vi "configure.vi"(8 "error in (no error)":errorcluster, 11 "DL090202ScanHead in":refnum<class "ScanHeadDL090202.lvclass">) -> (0 "error out":errorcluster, 3 "DL090202ScanHead out":refnum<class "ScanHeadDL090202.lvclass">)   [LabVIEW 2010, in "ScanHeadDL090202.lvclass"]
uses:
  ScanHeadDL090202.lvclass
  common/xcontrols/XComponentSpecification/XComponentSpecification/XComponentSpecification.xctl
  common/clusters/plugin_specification.ctl
  SignalWriter/GenericSignalWriter/GenericSignalWriter/GenericSignalWriter.lvclass
  ScanHeadDL090202.lvclass/ScanHeadDL090202.ctl
  Clock/GenericClock/GenericClock/GenericClock.lvclass
  DigitalOut/GenericDigitalOut/GenericDigitalOut/GenericDigitalOut.lvclass
  common/classes/ErrorController/ErrorController/class_data.vi
  common/classes/GenericComponent/GenericComponent/GenericComponent.lvclass
  common/classes/ErrorController/ErrorController/ErrorController.lvclass
panel:
  out "Configuration":string
  in  "cancel":bool
  in  "save":bool
  in  "Tab Control":T1(tab)=enum."shutter digital output"
  in  "x scanner factor":dbl[unit]=1000000.0 caption="translation factor"
  in  "y scanner factor":dbl[unit]=1000000.0 caption="translation factor"
  in  "z scanner factor":dbl[unit]=1000000.0 caption="translation factor"
  in  "xScanner spec":T2(xcontrol)
  in  "yScanner spec":T2(xcontrol)
  in  "zScanner spec":T2(xcontrol)
  in  "modifier factor":dbl=1.0 caption="translation factor"
  in  "intensity modified spec":T2(xcontrol)
  in  "clock spec":T2(xcontrol)
  in  "shutter digitalOut spec":T2(xcontrol)
  in  "offset Z":bool
  in  "offset Y":bool
  in  "offset X":bool
  in  "rotate Z":bool
  in  "zoom":bool
  in  "rotate X":bool
  # "Configure ScanHeadDL090202"
  # "SignalWriter components generate actuator values send to the scanners, each scanner has its own signal writer component.\n\nTranslation factors specify how the trajectory coordinates, which are defined in um space, are translated into the voltage values that are provided to the signalWriter component for each scanner."
  # "x scanner"
  # "y scanner"
  # "z scanner"
  # "Each pixel of the trajectory has a corresponding intensity value. Like the scanner values, the intensity control signal is generated by a SignalWriter component.\n\nThe translation factor specifies how an intensity value is translated into a voltage that is provided to the intensity modifier (such as a pockels cell).\nExample: 100% should correspond to 1.00V provided to a Pockels cell modulator; this would require the translation factor to be 0.01."
  # "The pixel clock is a Clock component that generates the TTL signal that is timingthe SignalWriter components generating the scanner and intensity modulator control signal."
  # "Here you can specify a software-controlled laser shutter. In case you are using an FPGA integrator, we recommend to use the shutter output of the Hifo ADC, because it is faster and more reliable. Leave empty in that case."
  # "Which user interface controls shall be visible?"
  # "For some sophisticated line-scan imagingModes, zooming and rotating etc. doesn't make sense, so the corresponding GUI controls should not be visible."
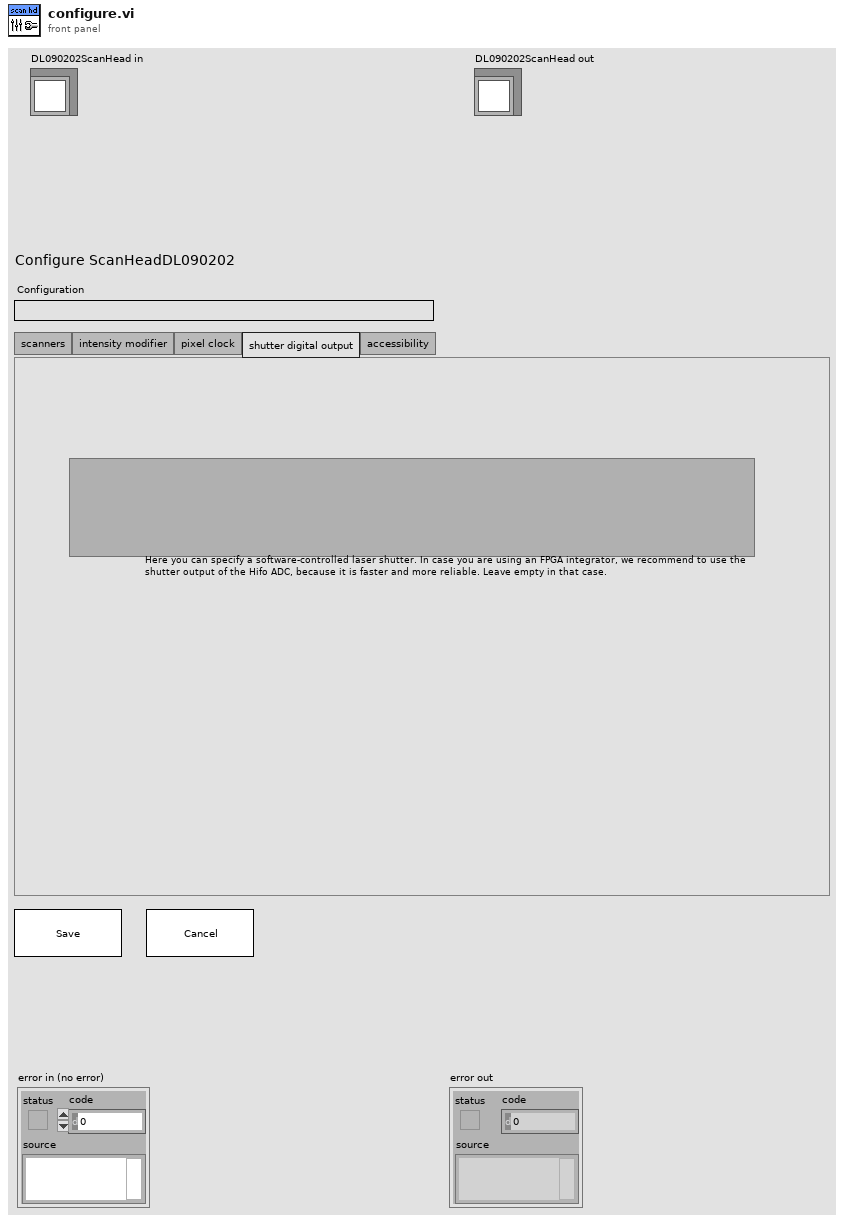
[diagram p1: front panel]
types:
  T1 = enum32{"scanners", "intensity modifier", "pixel clock", "shutter digital output", "accessibility"}
  T2 = cluster{"class path":string, "configuration":string, "label":string, "settings name":string}
  T3 = typedef "plugin_specification.ctl" = cluster{"class path":string, "configuration":string, "label":string, "settings name":string}
  T4 = cluster{"scanners[0]":T3, "scanners[1]":T3, "scanners[2]":T3}
  T5 = cluster{"scanner factors[0]":dbl[unit], "scanner factors[1]":dbl[unit], "scanner factors[2]":dbl[unit]}
  T6 = cluster{"class path":string, "configuration":string, "label":string, "settings name":string}[]
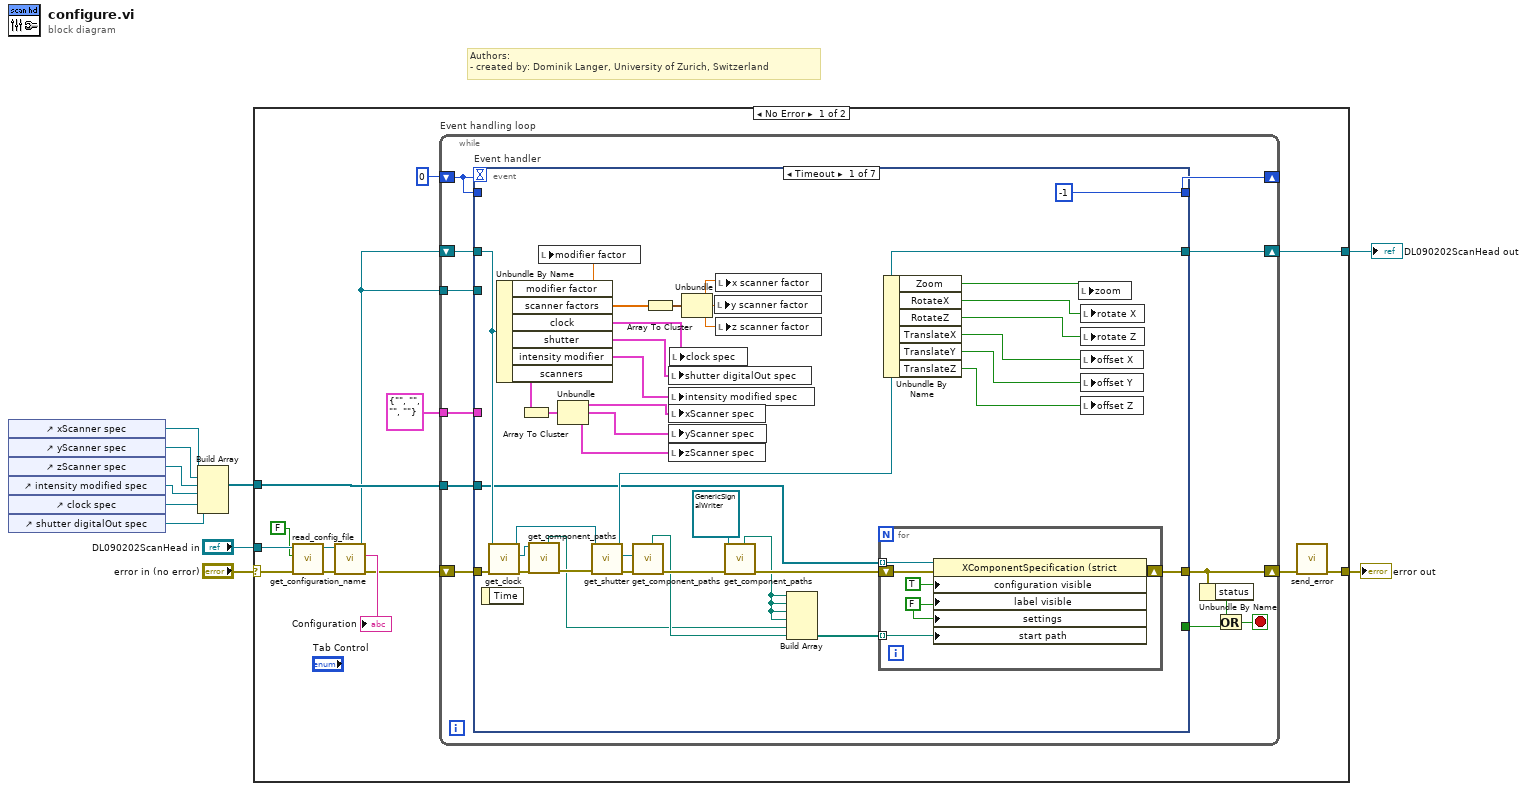
[diagram p0: block diagram]
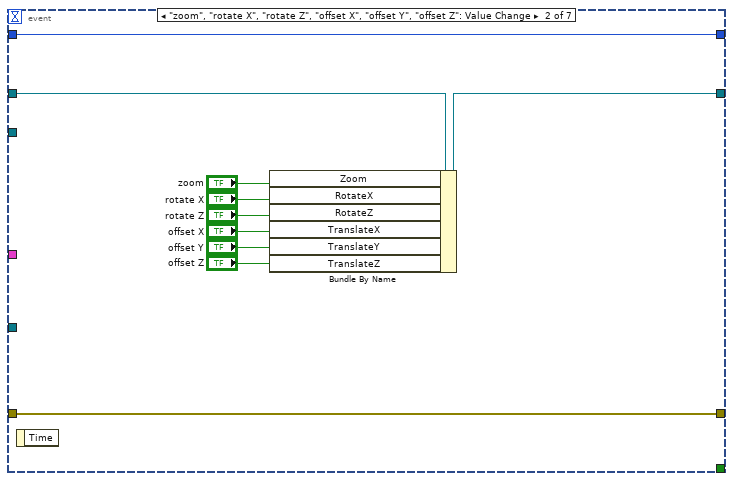
[diagram p2: hidden frame]
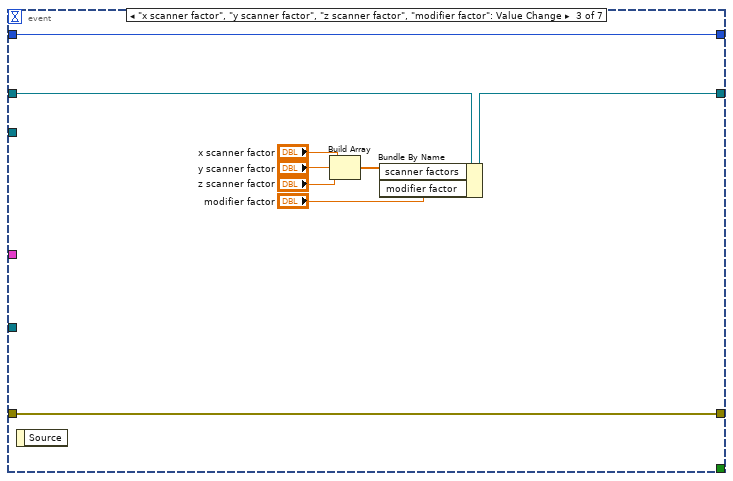
[diagram p3: hidden frame]
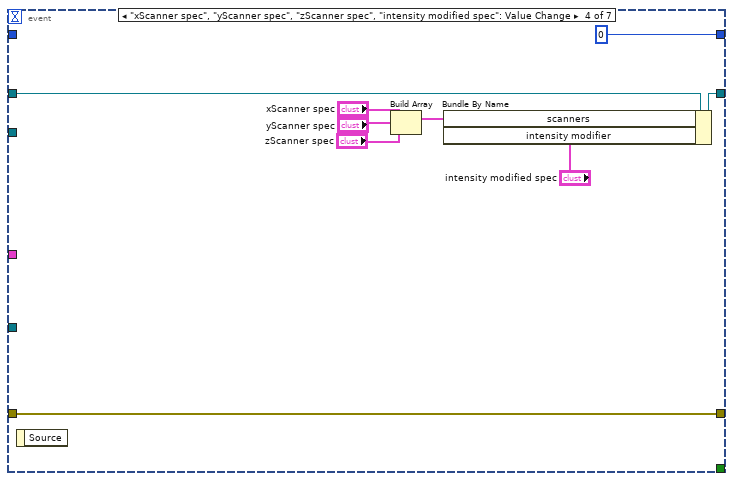
[diagram p4: hidden frame]
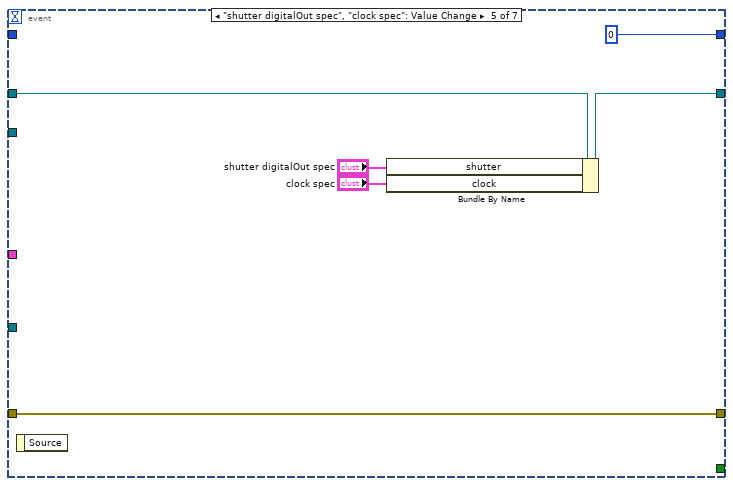
[diagram p5: hidden frame]
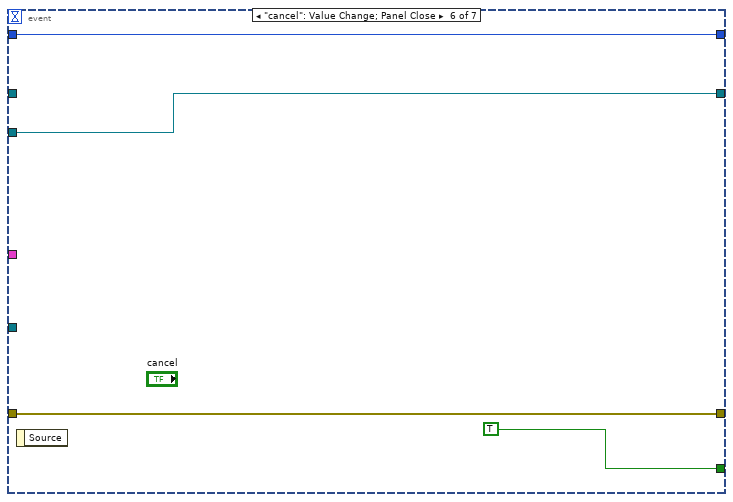
[diagram p6: hidden frame]
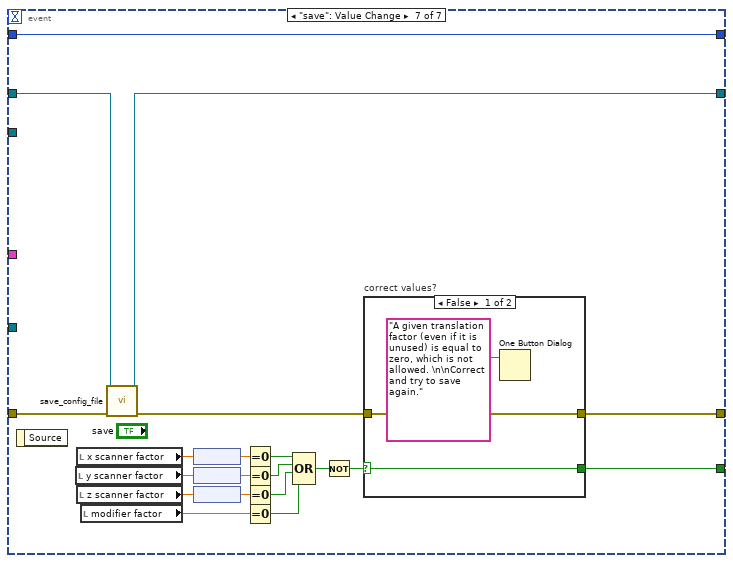
[diagram p7: hidden frame]
diagram:
  # "Authors: \n- created by: Dominik Langer, University of Zurich, Switzerland"
  n1 = control-ref of="xScanner spec"() -> (w6:refnum<vi>)
  n2 = control-ref of="yScanner spec"() -> (w5:refnum<vi>)
  n3 = control-ref of="zScanner spec"() -> (w4:refnum<vi>)
  n4 = control-ref of="intensity modified spec"() -> (w3:refnum<vi>)
  n5 = control-ref of="clock spec"() -> (w2:refnum<vi>)
  n6 = control-ref of="shutter digitalOut spec"() -> (w1:refnum<vi>)
  n7 = Build Array(w6, w5, w4, w3, w2, w1) -> (w8:refnum<vi>[])
  n8 = case shown="No Error" "error in (no error)" {
    selector: "error in (no error)" -> [w23 w147]
    tunnel: [w15 w147] -> w11
    tunnel: [w25 w146] -> w9
    tunnel: "DL090202ScanHead in" -> [w22 w146]
    tunnel: w8 -> [w21 _]
    frame No Error {
      n9 = call-dynamic "read_config_file.vi"("error in (no error)"=w23, "force load?"=FALSE, "GenericPlugin in"=w22) -> ("error out"=w12:errorcluster, "GenericPlugin out"=w19:refnum<class "ScanHeadDL090202.lvclass">)  [unwired: 7 out]
      n10 = call "get_configuration_name.vi"("error in (no error)"=w12, "GenericPlugin.lvclass in"=w19) -> ("error out"=w13:errorcluster, "configuration name"=→"Configuration":string, "GenericPlugin.lvclass out"=w16:refnum<class "ScanHeadDL090202.lvclass">)  [unwired: 7 in]
      n11 = while "Event handling loop" {
        shift-right: [w36] -> w25
        shift-left: w16 -> [w37]
        shift-right: [w34] -> _
        shift-left: 0 -> [w35]
        tunnel: w21 -> [w33]
        tunnel: T3 {"class path"="", "configuration"="", "label"="", "settings name"=""} ("configuration data.clock") -> [w32]
        tunnel: w16 -> [w31]
        shift-right: [w30] -> w14
        shift-left: w13 -> [w26]
        stop <- w28 stop-if-true
        n12 = event "Event handler" shown="[0] Timeout" {
          selector: _ -> [_ _ _ _ _ _ _]
          dyn-events: _ -> [_ _ _ _ _ _ _]
          timeout: w35 -> [_ _ _ _ _ _ _]
          tunnel: w26 -> [w62 w92 w101 w104 w113 w120 w138]
          tunnel: [w43 w92 w101 w104 w113 w120 w122] -> w30
          tunnel: [w55 w83 w99 w109 w114 w117 w139] -> w36
          tunnel: w37 -> [w56 w84 w94 w108 w115 _ w137]
          tunnel: [-1 w91 w100 0 0 w119 w140] -> w34
          tunnel: w35 -> [_ w91 w100 _ _ w119 w140]
          tunnel: [_ _ _ _ _ TRUE w123] -> w27
          tunnel: w33 -> [w38 _ _ _ _ _ _]
          tunnel: w32 -> [_ _ _ _ _ _ _]
          tunnel: w31 -> [_ _ _ _ _ w117 _]
          event Timeout {
            n13 = event-data() -> ()  [unwired: 2 out]
            n14 = call-dynamic "get_clock.vi"("error in (no error)"=w62, "DL090202ScanHead.lvclass in"=w56) -> ("error out"=w61:errorcluster, "GenericClock.lvclass"=w60:refnum<class "GenericClock.lvclass">, "DL090202ScanHead.lvclass out"=w57:refnum<class "ScanHeadDL090202.lvclass">)  [unwired: 7 in]
            n15 = Unbundle By Name(w56) -> ("modifier factor"=w63:dbl, "scanner factors"=w75:dbl[unit][], "clock"=w53:T3, "shutter"=w54:T3, "intensity modifier"=w52:T3, "scanners"=w50:T3[])
            n16 = Array To Cluster(array=w50) -> (cluster=w51:T4)
            n17 = call-dynamic "get_component_paths.vi"("error in (no error)"=w61, "GenericComponent in"=w60) -> ("error out"=w46:errorcluster, "component type directory"=w39:path)  [unwired: 4 in, 4 out]
            n18 = local write "modifier factor"(w63) -> ()
            n19 = Unbundle(w51) -> ("scanners[0]"=w49:T3, "scanners[1]"=w48:T3, "scanners[2]"=w47:T3)
            n20 = call-dynamic "get_shutter.vi"("error in (no error)"=w46, "DL090202ScanHead.lvclass in"=w57) -> ("error out"=w59:errorcluster, "GenericDigitalOut.lvclass"=w58:refnum<class "GenericDigitalOut.lvclass">, "DL090202ScanHead.lvclass out"=w55:refnum<class "ScanHeadDL090202.lvclass">)  [unwired: 7 in]
            n21 = call-dynamic "get_component_paths.vi"("error in (no error)"=w59, "GenericComponent in"=w58) -> ("error out"=w45:errorcluster, "component type directory"=w40:path)  [unwired: 4 in, 4 out]
            n22 = Array To Cluster(array=w75) -> (cluster=w76:T5)
            n23 = local write "shutter digitalOut spec"(w54) -> ()
            n24 = local write "intensity modified spec"(w52) -> ()
            n25 = local write "xScanner spec"(w49) -> ()
            n26 = local write "yScanner spec"(w48) -> ()
            n27 = local write "zScanner spec"(w47) -> ()
            n28 = local write "clock spec"(w53) -> ()
            n29 = Unbundle(w76) -> ("scanner factors[0]"=w74:dbl[unit], "scanner factors[1]"=w73:dbl[unit], "scanner factors[2]"=w72:dbl[unit])
            n30 = local write "y scanner factor"(w73) -> ()
            n31 = local write "x scanner factor"(w74) -> ()
            n32 = local write "z scanner factor"(w72) -> ()
            n33 = call-dynamic "get_component_paths.vi"("error in (no error)"=w45, "GenericComponent in"=refnum<class "GenericSignalWriter.lvclass"> refnum ("GenericSignalWriter.lvclass")) -> ("error out"=w44:errorcluster, "component type directory"=w42:path)  [unwired: 4 in, 4 out]
            n34 = Build Array(w42, w42, w42, w42, w39, w40) -> (w41:path[])
            n35 = for {
              shift-right: [w79] -> w43
              shift-left: w44 -> [w80]
              tunnel: w41 -> [w78] mode=indexing
              tunnel: w38 -> [w77] mode=indexing
              w81 = FALSE ("configuration visible")
              n36 = property on="Property Node" class="XComponentSpecification (strict"(reference=w77, error in=w80, "configuration visible"=TRUE, "label visible"=w81, "settings"=w81, "start path"=w78) -> (error out=w79:errorcluster)  [unwired: 1 out]
            }
            n37 = Unbundle By Name(w55) -> ("Zoom"=w70:bool, "RotateX"=w69:bool, "RotateZ"=w68:bool, "TranslateX"=w67:bool, "TranslateY"=w66:bool, "TranslateZ"=w65:bool)
            n38 = local write "zoom"(w70) -> ()
            n39 = local write "rotate X"(w69) -> ()
            n40 = local write "rotate Z"(w68) -> ()
            n41 = local write "offset X"(w67) -> ()
            n42 = local write "offset Y"(w66) -> ()
            n43 = local write "offset Z"(w65) -> ()
          }
          event "zoom", "rotate X", "rotate Z", "offset X", "offset Y", "offset Z": Value Change {
            n44 = event-data() -> ()  [unwired: 2 out]
            n45 = Bundle By Name(cluster=w84, "Zoom"="zoom", "RotateX"="rotate X", "RotateZ"="rotate Z", "TranslateX"="offset X", "TranslateY"="offset Y", "TranslateZ"="offset Z") -> (w83:refnum<class "ScanHeadDL090202.lvclass">)
          }
          event "x scanner factor", "y scanner factor", "z scanner factor", "modifier factor": Value Change {
            n46 = event-data() -> ()  [unwired: 2 out]
            n47 = Build Array("x scanner factor", "y scanner factor", "z scanner factor") -> (w95:dbl[unit][])
            n48 = Bundle By Name(cluster=w94, "scanner factors"=w95, "modifier factor"="modifier factor") -> (w99:refnum<class "ScanHeadDL090202.lvclass">)
          }
          event "xScanner spec", "yScanner spec", "zScanner spec", "intensity modified spec": Value Change {
            n49 = event-data() -> ()  [unwired: 2 out]
            n50 = Build Array("xScanner spec", "yScanner spec", "zScanner spec") -> (w110:T6)
            n51 = Bundle By Name(cluster=w108, "scanners"=w110, "intensity modifier"="intensity modified spec") -> (w109:refnum<class "ScanHeadDL090202.lvclass">)
          }
          event "shutter digitalOut spec", "clock spec": Value Change {
            n52 = event-data() -> ()  [unwired: 2 out]
            n53 = Bundle By Name(cluster=w115, "shutter"="shutter digitalOut spec", "clock"="clock spec") -> (w114:refnum<class "ScanHeadDL090202.lvclass">)
          }
          event "cancel": Value Change; Panel Close {
            n54 = event-data() -> ()  [unwired: 2 out]
          }
          event "save": Value Change {
            n55 = event-data() -> ()  [unwired: 2 out]
            n56 = local read "y scanner factor"() -> (w134:dbl[unit])
            n57 = local read "x scanner factor"() -> (w136:dbl[unit])
            n58 = local read "z scanner factor"() -> (w133:dbl[unit])
            n59 = local read "modifier factor"() -> (w132:dbl)
            n60 = call-dynamic "save_config_file.vi"("error in (no error)"=w138, "GenericPlugin in"=w137) -> ("error out"=w121:errorcluster, "GenericPlugin out"=w139:refnum<class "ScanHeadDL090202.lvclass">)  [unwired: 2 in, 6 out]
            n61 = node(w136) -> (w135:dbl)
            n62 = node(w134) -> (w130:dbl)
            n63 = node(w133) -> (w131:dbl)
            n64 = Equal To 0?(x=w135) -> (x = 0?=w129:bool)
            n65 = Equal To 0?(x=w130) -> (x = 0?=w128:bool)
            n66 = Equal To 0?(x=w131) -> (x = 0?=w127:bool)
            n67 = Equal To 0?(x=w132) -> (x = 0?=w126:bool)
            n68 = Compound Arithmetic op=OR(w129, w128, w127, w126) -> (w125:bool)
            n69 = Not(x=w125) -> (.not. x?=w124:bool)
            n70 = case "correct values?" shown="False" w124 {
              selector: w124 -> [w143 w145]
              tunnel: [w143 w145] -> w123
              tunnel: [w142 w144] -> w122
              tunnel: w121 -> [w142 w144]
              frame False {
                n71 = One Button Dialog(message="A given translation factor (even if it is unused) is equal to zero, which is not allowed. \n\nCorrect and try to save again.") -> ()  [unwired: 1 in, 1 out]
              }
              frame True {
              }
            }
          }
        }
        n72 = Unbundle By Name(w30) -> ("status"=w29:bool)
        n73 = Or(x=w29, y=w27) -> (x .or. y?=w28:bool)
      }
      n74 = call "send_error.vi"("error in (no error)"=w14) -> ("error out"=w15:errorcluster)  [unwired: 10 in]
    }
    frame Error {
    }
  }
  "error out" <- w11
  "DL090202ScanHead out" <- w9
